vi "parameterized_SessionInitializeErrors_InitializeSessions_CloseCalledForPreviouslyInitializedSessionsWithProperBehavior.vi"(0 "expected initialize-initialize calls":u32, 1 "initialize and close session behavior":T1, 5 "expected initialize-attach calls":u32, 7 "expected close-close calls":u32, 9 "expected close-detach calls":u32, 11 "error in":errorcluster) -> (4 "pass":bool, 6 "result":string, 15 "error out":errorcluster)   [LabVIEW 2020, in "MeasurementServerTests.lvlib"]
uses:
  MeasurementServerTests.lvlib
  Runtime/MeasurementLink Session Management/Session Reservation/Initialize and Close Session Behavior.ctl
  da6ffb6f-c1c9-4957-84dd-e9228483c454.vi
  ffc64c76-1568-41a3-8328-b9126ac9a28d.vi
  Helpers/Fake Session Factory/Fake Session Factory.lvclass
  C:/dev/measurementlink-labview/Source/Runtime/MeasurementLink Instrument/ISession Factory/ISession Factory.lvclass
  Runtime/MeasurementLink Session Management/Session Reservation/Initialize Sessions with Retry.vi
  Runtime/MeasurementLink Session Management/Session Reservation/Session Reservation.lvclass
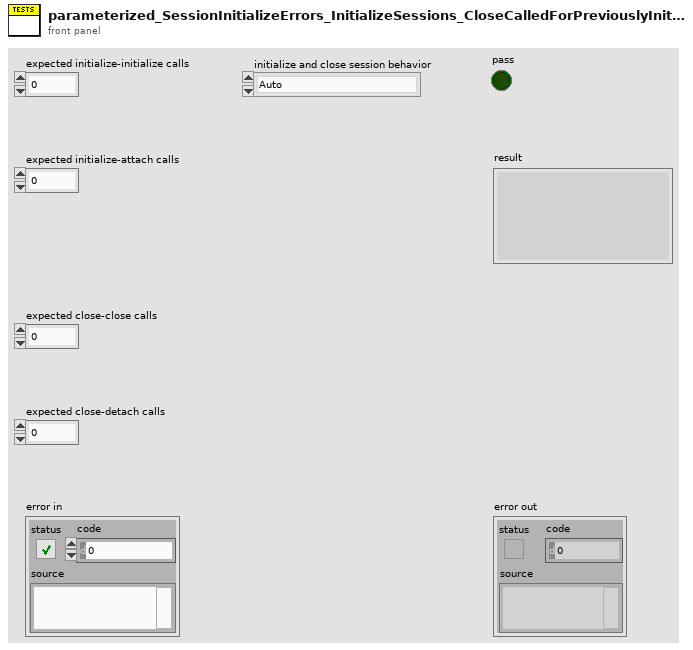
[diagram p1: front panel]
types:
  T1 = typedef "MeasurementLink Session Management.lvlib/Session Reservation.lvclass/Initialize and Close Session Behavior.ctl" = enum16{"Auto", "Initialize and Close", "Attach and Detach", "Initialize and Detach", "Attach and Close"}
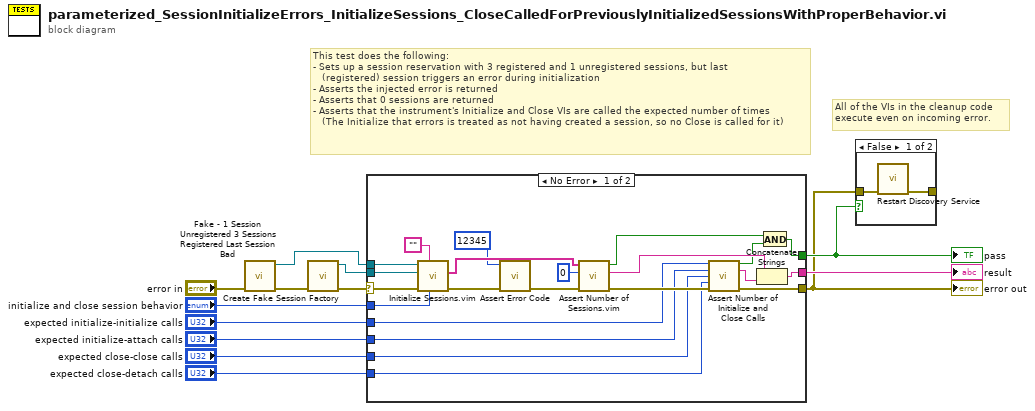
[diagram p0: block diagram]
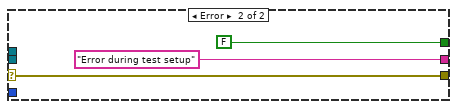
[diagram p2: hidden frame]
diagram:
  # "All of the VIs in the cleanup code\nexecute even on incoming error."
  # "This test does the following:\n- Sets up a session reservation with 3 registered and 1 unregistered sessions, but last\n   (registered) session triggers an error during initialization\n- Asserts the injected error is returned\n- Asserts that 0 sessions are returned\n- Asserts that the instrument's Initialize and Close VIs are called the expected number of times\n   (The Initialize that errors is treated as not having created a session, so no Close is called for it)"
  n1 = call "Fake - 1 Session Unregistered 3 Sessions Registered Last Session Bad.vi"("error in"="error in") -> ("error out"=w7:errorcluster, "session reservation out"=w6:refnum<class "Session Reservation.lvclass">)  [unwired: 9 in]
  n2 = call "Create Fake Session Factory.vi"("error in"=w7) -> ("error out"=w10:errorcluster, "fake session factory out"=w9:refnum<class "Fake Session Factory.lvclass">)  [unwired: 9 in]
  n3 = case shown="No Error" w10 {
    selector: w10 -> [w33 w36]
    tunnel: [w25 w36] -> w11
    tunnel: [w24 FALSE] -> w12
    tunnel: [w22 "Error during test setup" ("f")] -> w13
    tunnel: w9 -> [w35 _]
    tunnel: w6 -> [w34 _]
    tunnel: "initialize and close session behavior" -> [w18 _]
    tunnel: "expected initialize-initialize calls" -> [w17 _]
    tunnel: "expected initialize-attach calls" -> [w16 _]
    tunnel: "expected close-close calls" -> [w15 _]
    tunnel: "expected close-detach calls" -> [w14 _]
    frame No Error {
      n4 = call "Initialize Sessions.vim"("initialize and close session behavior"=w18, "session type"="", "error in"=w33, "session factory"=w35, "session reservation in"=w34) -> ("error out"=w32:errorcluster, "sessions"=w30:string[])  [unwired: 3 in, 2 out]
      n5 = call "Assert Error Code.vi"("error in"=w32, "expected error code"=12345) -> ("error out"=w20:errorcluster)  [unwired: 7 in, 2 out]
      n6 = call "Assert Number of Sessions.vim"("error in"=w20, "expected number of sessions"=0, "sessions"=w30) -> ("error out"=w26:errorcluster, "result"=w29:string, "pass"=w28:bool)  [unwired: 6 in]
      n7 = call "Assert Number of Initialize and Close Calls.vi"("expected initialize-initialize calls"=w17, "expected initialize-attach calls"=w16, "expected close-close calls"=w15, "expected close-detach calls"=w14, "error in"=w26) -> ("pass"=w23:bool, "result"=w21:string, "error out"=w25:errorcluster)  [unwired: 8 in]
      n8 = Concatenate Strings(w29, w21) -> (w22:string)
      n9 = And(x=w28, y=w23) -> (x .and. y?=w24:bool)
    }
    frame Error {
    }
  }
  "error out" <- w11
  "pass" <- w12
  "result" <- w13
  n10 = case shown="False" w12 {
    tunnel: w11 -> [w40 _]
    tunnel: [w39 _] -> _
    frame False {
      n11 = call "Restart Discovery Service.vi"("error in"=w40) -> ("error out"=w39:errorcluster)  [unwired: 10 in]
    }
    frame True {
    }
  }
